vi "Write Duration.vi"(10 "Duration":i32 format="%<%H:%M:%S>t", 11 "RetentionPolicy in":refnum<class "RetentionPolicy.lvclass">) -> (3 "RetentionPolicy out":refnum<class "RetentionPolicy.lvclass">)   [LabVIEW 2018, in "InfluxDB Client.lvlib" / "RetentionPolicy.lvclass"]
uses:
  RetentionPolicy.lvclass
  RetentionPolicy.lvclass/RetentionPolicy.ctl
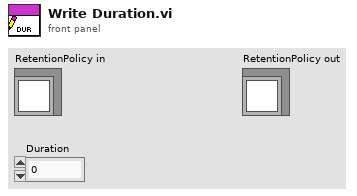
[diagram p1: front panel]
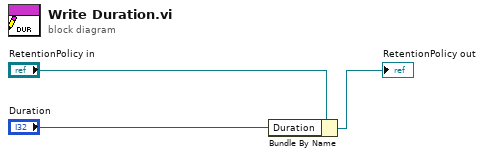
[diagram p0: block diagram]
diagram:
  n1 = Bundle By Name(cluster="RetentionPolicy in", "Duration"="Duration") -> (→"RetentionPolicy out":refnum<class "RetentionPolicy.lvclass">)
